vi "AMI_CREA_SECUENCIA_REPITE.vi"(8 "error in (no error)":errorcluster) -> (0 "error out":errorcluster, 1 "Total":string[](array[string]), 2 "Pasos":i32, 3 "Secuencia":string[](array[string]), 4 "Secuciclos":string[](array[string]), 6 "Pasos f":i32)   [LabVIEW 2017]
uses:
  <vilib>/Utility/file.llb/Read Delimited Spreadsheet (string).vi
panel:
  out "idxScanXi":i16
  out "idxScanXf":i16
  out "idxScanYi":i16
  out "idxScanYf":i16
  out "Scan X":bool
  out "Scan Y":bool
  out "idxScanVi":i16
  out "idxScanVf":i16
  out "Scan V":bool
  out "subArray2D":string[][](array[string])
  out "Seq scans":string[](array[string])
  out "Seq final":string[](array[string])
  out "Seq inicial":string[](array[string])
  out "idxScanTi":i16
  out "idxScanZi":i16
  out "idxScanZf":i16
  out "idxScanTf":i16
  out "Array2D":string[][](array[string])
  out "Scan T":bool
  out "Scan Z":bool
  in  "Salir":bool
  in  "Borrar línea":bool
  in  "Grabar":bool
  in  "Cargar":bool
  out "SequenceFile":path
  in  "Añadir: (doble click)":i32(listbox) caption="Válvulas"
  in  "Secuencia":i32(listbox)=-1
  # "Nov 2022 V1.6  a-sslcdms"
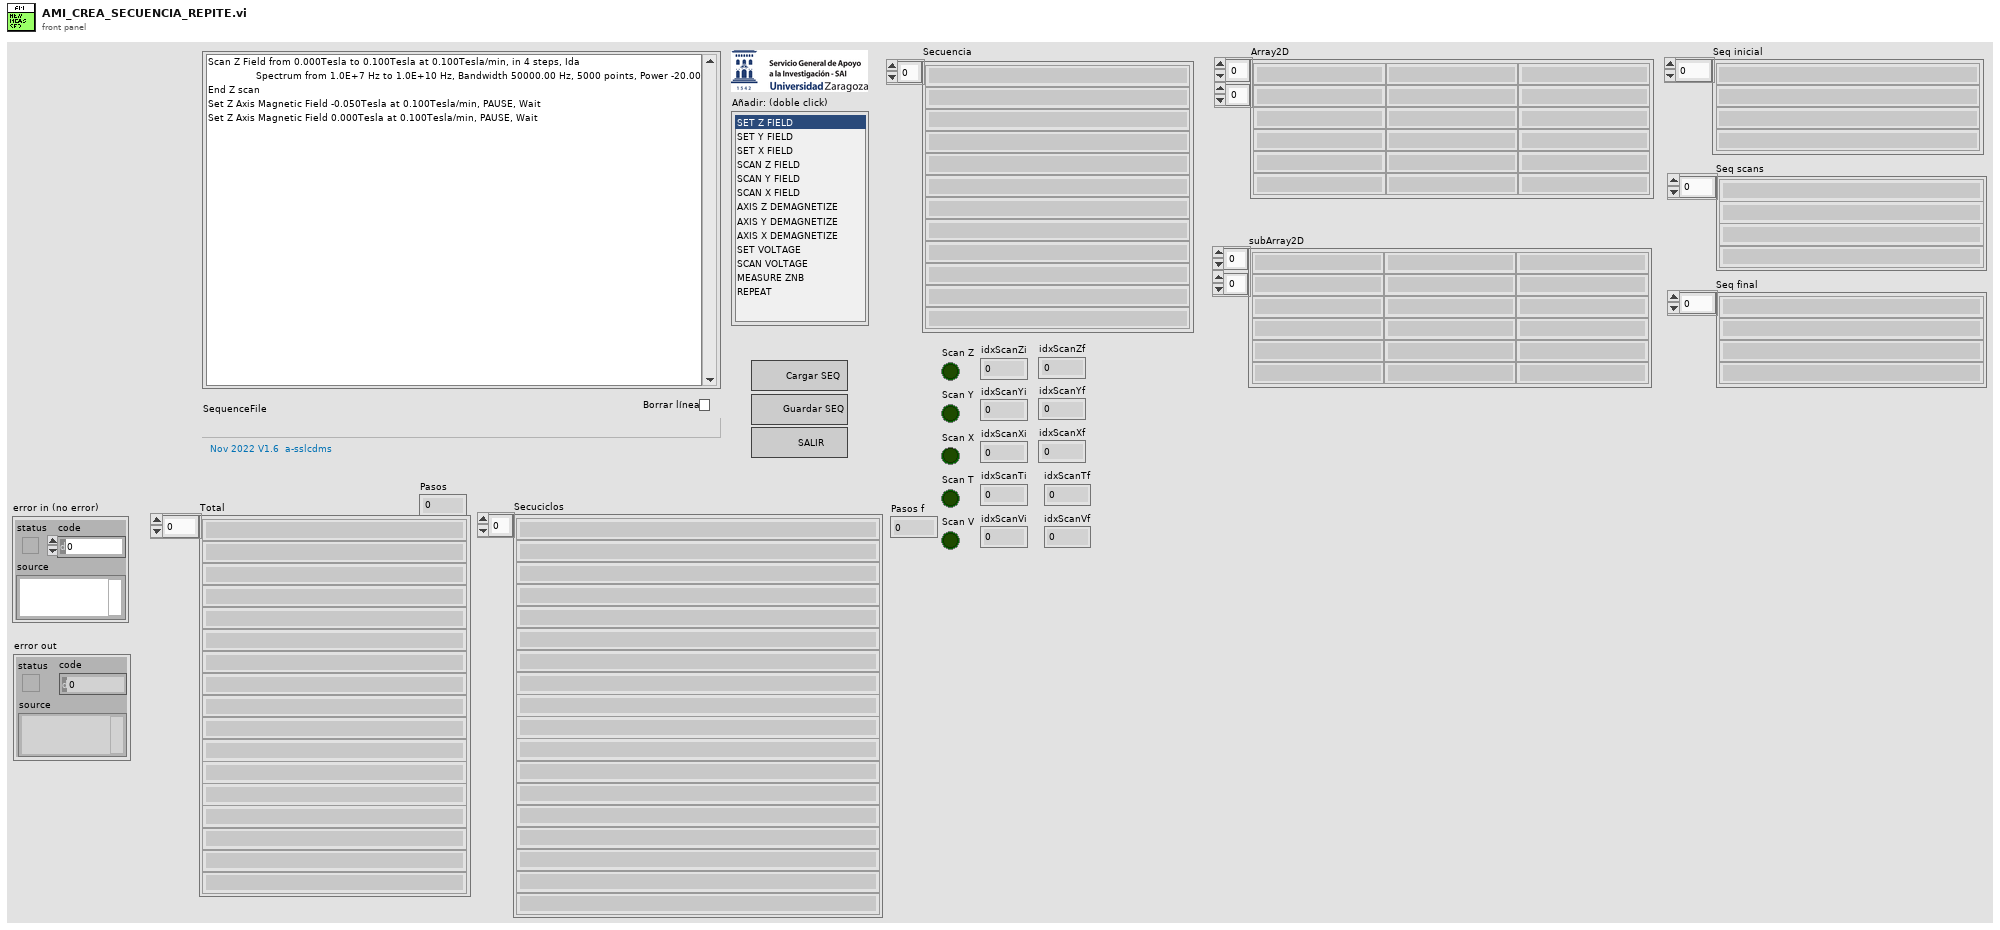
[diagram p1: front panel]
types:
  T1 = enum16{"open", "open or create", "create or replace", "create", "open (read only)"}
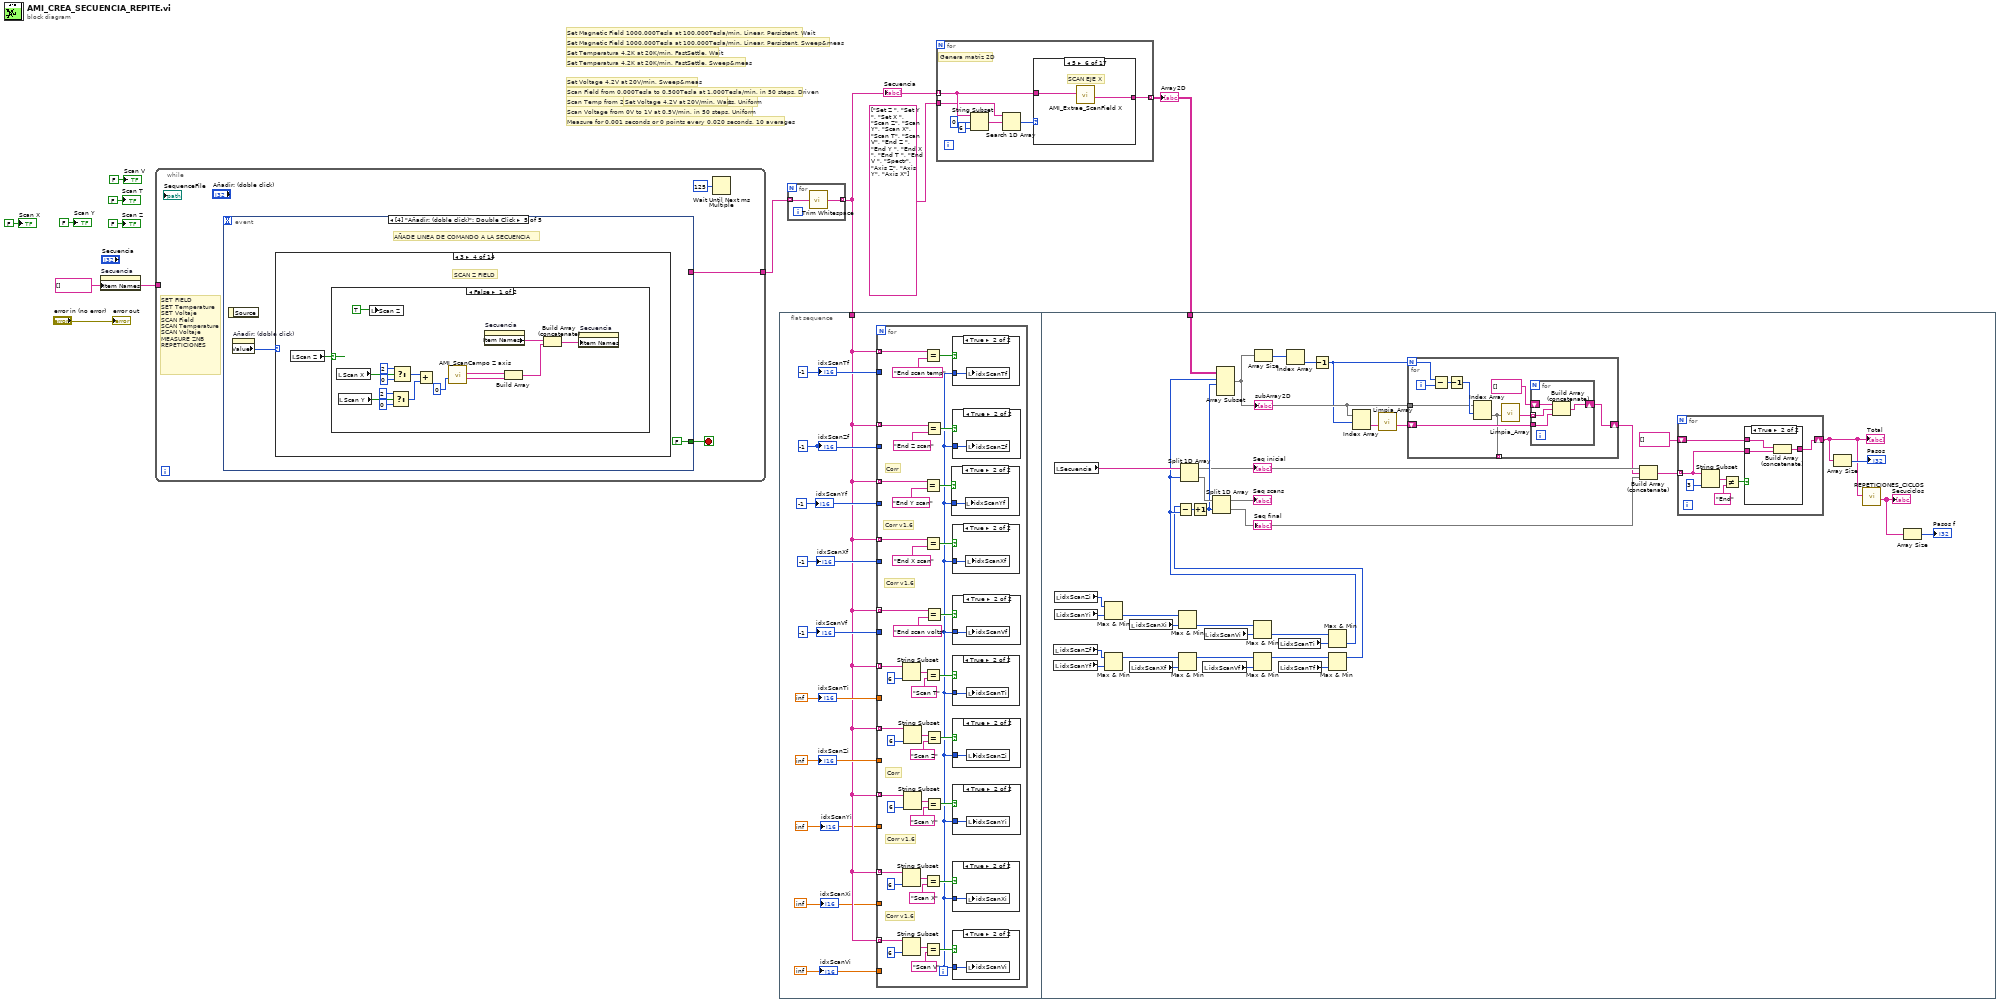
[diagram p0: block diagram]
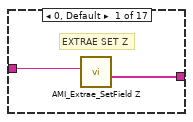
[diagram p13: hidden frame]
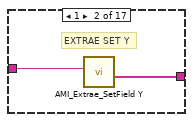
[diagram p14: hidden frame]
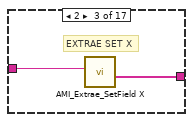
[diagram p15: hidden frame]
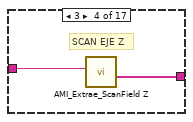
[diagram p16: hidden frame]
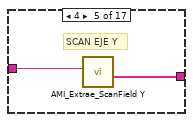
[diagram p17: hidden frame]
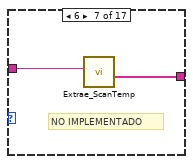
[diagram p18: hidden frame]
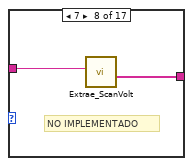
[diagram p19: hidden frame]
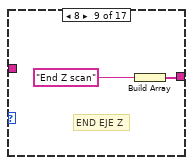
[diagram p20: hidden frame]
diagram:
  w11 = string[] [] ("Item Names")
  # "Measure for 0.001 seconds or 0 points every 0.020 seconds, 10 averages"
  # "Scan Voltage from 0V to 1V at 0.5V/min, in 50 steps, Uniform"
  # "Scan Temp from 20K to 200K at 0.1K/min, in 50 steps, Uniform"
  # "Scan Field from 0.000Tesla to 0.500Tesla at 1.000Tesla/min, in 50 steps, Driven"
  # "Set Temperatura 4.2K at 20K/min, FastSettle, Sweep&meas"
  # "Set Temperatura 4.2K at 20K/min, FastSettle, Wait"
  # "Set Magnetic Field 1000.000Tesla at 100.000Tesla/min, Linear, Persistent, Sweep&meas"
  # "Set Magnetic Field 1000.000Tesla at 100.000Tesla/min, Linear, Persistent, Wait"
  # "Set Voltage 4.2V at 20V/min, Sweep&meas"
  # "Set Voltage 4.2V at 20V/min, Wait"
  n1 = property on="Secuencia" class="LstBox (strict)"("Item Names"=w11) -> ()  [unwired: 2 in, 2 out]
  n2 = while {
    tunnel: w11 -> [_]
    tunnel: [w12] -> w6
    stop <- w13 stop-if-true
    # "SET FIELD\nSET Temperature\nSET Voltaje\nSCAN Field\nSCAN Temperature\nSCAN Voltaje\nMEASURE ZNB\nREPETICIONES"
    n3 = event shown="[4] \"Añadir: (doble click)\": Double Click" {
      selector: _ -> [_ _ _ _ _]
      dyn-events: _ -> [_ _ _ _ _]
      timeout: _ -> [_ _ _ _ _]
      tunnel: [FALSE ("Salir") "Salir" FALSE ("Salir") FALSE ("Salir") FALSE ("Salir")] -> w13
      tunnel: [_ w20 _ _ _] -> w12
      event "Borrar línea": Value Change {
        # "BORRA LA LINEA ACTIVA DE LA SECUENCIA"
        n4 = event-data() -> ()  [unwired: 1 in, 1 out]
        n5 = property on="Secuencia" class="LstBox (strict)"() -> ("Item Names"=w19:string[], "Value"=w18:i32)  [unwired: 2 in, 2 out]
        n6 = Delete From Array(array=w19, length=1, index=w18) -> (array with subset deleted=w16:string[])  [unwired: 1 out]
        n7 = property on="Secuencia" class="LstBox (strict)"("Item Names"=w16) -> ()  [unwired: 2 in, 2 out]
      }
      event "Salir": Value Change {
        # "SALIMOS DEL VI"
        n8 = event-data() -> ()  [unwired: 1 in, 1 out]
        n9 = property on="Secuencia" class="LstBox (strict)"() -> ("Item Names"=w20:string[])  [unwired: 2 in, 2 out]
      }
      event "Cargar": Value Change {
        # "CARGA UNA SECUENCIA ALMACENADA PREVIAMENTE"
        n10 = event-data() -> ()  [unwired: 1 in, 1 out]
        n11 = call-poly <vilib>:"Read Delimited Spreadsheet.vi"() -> ("new file path (Not A Path if cancelled)"=w23:path, "all rows"=w22:string[][])  [unwired: 10 in, 4 out]
        n12 = local write "SequenceFile"(w23) -> ()
        n13 = Index Array(array=w22, index (col)=0 ("disabled index (col)")) -> (element=w24:string[])  [unwired: 1 in]
        n14 = property on="Secuencia" class="LstBox (strict)"("Item Names"=w24) -> ()  [unwired: 2 in, 2 out]
      }
      event "Grabar": Value Change {
        # "GRABA UNA SECUENCIA PARA USAR MAS ADELANTE"
        n15 = event-data() -> ()  [unwired: 1 in, 1 out]
        n16 = property on="Secuencia" class="LstBox (strict)"() -> ("Item Names"=w30:string[])  [unwired: 2 in, 2 out]
        n17 = call <vilib>:"Open_Create_Replace File.vi"("function (open:0)"=T1."create or replace") -> ("new file path"=w27:path)  [unwired: 7 in, 3 out]
        n18 = local write "SequenceFile"(w27) -> ()
        n19 = for {
          tunnel: w30 -> [w33] mode=indexing
          shift-right: [w35] -> _
          shift-left: w27 -> [w36]
          n20 = Concatenate Strings(w33, "\r\n") -> (w32:string)
          n21 = call <vilib>:"Write Characters To File.vi"("append to file? (new file:F)"=TRUE, "character string"=w32, "file path (dialog if empty)"=w36) -> ("new file path (Not A Path if cancelled)"=w35:path)  [unwired: 2 in]
        }
      }
      event "Añadir: (doble click)": Double Click {
        # "AÑADE LINEA DE COMANDO A LA SECUENCIA"
        n22 = event-data() -> ()  [unwired: 1 in, 1 out]
        n23 = property on="Añadir: (doble click)" class="LstBox (strict)"() -> ("Value"=w37:i32)  [unwired: 2 in, 2 out]
        n24 = case shown="3" w37 {
          frame 0, Default {
            # "SET Z FIELD"
            n25 = property on="Secuencia" class="LstBox (strict)"() -> ("Item Names"=w39:string[])  [unwired: 2 in, 2 out]
            n26 = call "AMI_SetCampo Z axis.vi"("Index"=i8 0) -> ("resulting string Z"=w41:string)  [unwired: 7 in, 1 out]
            n27 = Build Array (concatenate)(w39, w41) -> (w40:string[])
            n28 = property on="Secuencia" class="LstBox (strict)"("Item Names"=w40) -> ()  [unwired: 2 in, 2 out]
          }
          frame 1 {
            # "SET Y FIELD"
            n29 = property on="Secuencia" class="LstBox (strict)"() -> ("Item Names"=w44:string[])  [unwired: 2 in, 2 out]
            n30 = call "AMI_SetCampo Y axis.vi"("Index"=i8 0) -> ("resulting string Y"=w46:string)  [unwired: 7 in, 1 out]
            n31 = Build Array (concatenate)(w44, w46) -> (w45:string[])
            n32 = property on="Secuencia" class="LstBox (strict)"("Item Names"=w45) -> ()  [unwired: 2 in, 2 out]
          }
          frame 2 {
            # "SET X FIELD"
            n33 = property on="Secuencia" class="LstBox (strict)"() -> ("Item Names"=w50:string[])  [unwired: 2 in, 2 out]
            n34 = call "AMI_SetCampo X axis.vi"("Index"=i8 0) -> ("resulting string X"=w48:string)  [unwired: 7 in, 1 out]
            n35 = Build Array (concatenate)(w50, w48) -> (w49:string[])
            n36 = property on="Secuencia" class="LstBox (strict)"("Item Names"=w49) -> ()  [unwired: 2 in, 2 out]
          }
          frame 3 {
            # "SCAN Z FIELD"
            n37 = local read "Scan Z"() -> (w51:bool)
            n38 = case shown="False" w51 {
              frame False {
                n39 = local read "Scan X"() -> (w63:bool)
                n40 = local read "Scan Y"() -> (w62:bool)
                n41 = local write "Scan Z"(TRUE ("Scan T")) -> ()
                n42 = Select(t=i8 2 ("Index"), s=w62, f=i8 0 ("Index")) -> (s? t:f=w58:i8)
                n43 = Select(t=i8 2 ("Index"), s=w63, f=i8 0 ("Index")) -> (s? t:f=w59:i8)
                n44 = Add(x=w59, y=w58) -> ()  [unwired: 1 out]
                n45 = call "AMI_ScanCampo Z axis.vi"("Index"=i8 0) -> ("resulting string 2"=w53:string, "resulting string 1"=w52:string)  [unwired: 6 in, 1 out]
                n46 = property on="Secuencia" class="LstBox (strict)"() -> ("Item Names"=w56:string[])  [unwired: 2 in, 2 out]
                n47 = Build Array(w52, w53) -> (w55:string[])
                n48 = Build Array (concatenate)(w56, w55) -> (w54:string[])
                n49 = property on="Secuencia" class="LstBox (strict)"("Item Names"=w54) -> ()  [unwired: 2 in, 2 out]
              }
              frame True {
                n50 = One Button Dialog(message="Solo esta permitido\nun scan de campo por secuencia") -> ()  [unwired: 1 in, 1 out]
              }
            }
          }
          frame 4 {
            # "SCAN Y FIELD"
            n51 = local read "Scan Y"() -> (w68:bool)
            n52 = case shown="False" w68 {
              frame False {
                n53 = local read "Scan X"() -> (w80:bool)
                n54 = local read "Scan Z"() -> (w79:bool)
                n55 = local write "Scan Y"(TRUE ("Scan T")) -> ()
                n56 = Select(t=i8 2 ("Index"), s=w79, f=i8 0 ("Index")) -> (s? t:f=w75:i8)
                n57 = Select(t=i8 2 ("Index"), s=w80, f=i8 0 ("Index")) -> (s? t:f=w76:i8)
                n58 = Add(x=w76, y=w75) -> ()  [unwired: 1 out]
                n59 = call "AMI_ScanCampo Y axis.vi"("Index"=i8 0) -> ("resulting string 2"=w70:string, "resulting string 1"=w69:string)  [unwired: 6 in, 1 out]
                n60 = property on="Secuencia" class="LstBox (strict)"() -> ("Item Names"=w73:string[])  [unwired: 2 in, 2 out]
                n61 = Build Array(w69, w70) -> (w72:string[])
                n62 = Build Array (concatenate)(w73, w72) -> (w71:string[])
                n63 = property on="Secuencia" class="LstBox (strict)"("Item Names"=w71) -> ()  [unwired: 2 in, 2 out]
              }
              frame True {
                n64 = One Button Dialog(message="Solo esta permitido\nun scan de campo por secuencia") -> ()  [unwired: 1 in, 1 out]
              }
            }
          }
          frame 5 {
            # "SCAN X FIELD"
            n65 = local read "Scan X"() -> (w85:bool)
            n66 = case shown="False" w85 {
              frame False {
                n67 = local read "Scan Y"() -> (w97:bool)
                n68 = local read "Scan Z"() -> (w96:bool)
                n69 = local write "Scan X"(TRUE ("Scan T")) -> ()
                n70 = Select(t=i8 2 ("Index"), s=w96, f=i8 0 ("Index")) -> (s? t:f=w92:i8)
                n71 = Select(t=i8 2 ("Index"), s=w97, f=i8 0 ("Index")) -> (s? t:f=w93:i8)
                n72 = Add(x=w93, y=w92) -> ()  [unwired: 1 out]
                n73 = call "AMI_ScanCampo X axis.vi"("Index"=i8 0) -> ("resulting string 2"=w87:string, "resulting string 1"=w86:string)  [unwired: 6 in, 1 out]
                n74 = property on="Secuencia" class="LstBox (strict)"() -> ("Item Names"=w90:string[])  [unwired: 2 in, 2 out]
                n75 = Build Array(w86, w87) -> (w89:string[])
                n76 = Build Array (concatenate)(w90, w89) -> (w88:string[])
                n77 = property on="Secuencia" class="LstBox (strict)"("Item Names"=w88) -> ()  [unwired: 2 in, 2 out]
              }
              frame True {
                n78 = One Button Dialog(message="Solo esta permitido\nun scan de campo por secuencia") -> ()  [unwired: 1 in, 1 out]
              }
            }
          }
          frame 6 {
            # "DESIMANAR Z FIELD"
            n79 = property on="Secuencia" class="LstBox (strict)"() -> ("Item Names"=w102:string[])  [unwired: 2 in, 2 out]
            n80 = call "AMI_Desimana Z axis.vi"("Index"=i8 0) -> ("resulting string Z"=w104:string)  [unwired: 7 in, 1 out]
            n81 = Build Array (concatenate)(w102, w104) -> (w103:string[])
            n82 = property on="Secuencia" class="LstBox (strict)"("Item Names"=w103) -> ()  [unwired: 2 in, 2 out]
          }
          frame 7 {
            # "DESIMANAR Y FIELD"
            n83 = property on="Secuencia" class="LstBox (strict)"() -> ("Item Names"=w107:string[])  [unwired: 2 in, 2 out]
            n84 = call "AMI_Desimana Y axis.vi"("Index"=i8 0) -> ("resulting string Y"=w109:string)  [unwired: 7 in, 1 out]
            n85 = Build Array (concatenate)(w107, w109) -> (w108:string[])
            n86 = property on="Secuencia" class="LstBox (strict)"("Item Names"=w108) -> ()  [unwired: 2 in, 2 out]
          }
          frame 8 {
            # "DESIMANAR X FIELD"
            n87 = property on="Secuencia" class="LstBox (strict)"() -> ("Item Names"=w113:string[])  [unwired: 2 in, 2 out]
            n88 = call "AMI_Desimana X axis.vi"("Index"=i8 0) -> ("resulting string X"=w111:string)  [unwired: 7 in, 1 out]
            n89 = Build Array (concatenate)(w113, w111) -> (w112:string[])
            n90 = property on="Secuencia" class="LstBox (strict)"("Item Names"=w112) -> ()  [unwired: 2 in, 2 out]
          }
          frame 9 {
            # "SET VOLTAGE"
            n91 = case shown="False" FALSE {
              frame False {
                n92 = One Button Dialog(message="Comando desactivado") -> ()  [unwired: 1 in, 1 out]
              }
              frame True {
                n93 = call "PPMS_SetVoltage.vi"("Index"=i8 0) -> ("resulting string 1"=w117:string, "Cancelled?"=w118:bool)  [unwired: 6 in, 1 out]
                n94 = case shown="False" w118 {
                  tunnel: w117 -> [w121 _]
                  frame False {
                    n95 = property on="Secuencia" class="LstBox (strict)"() -> ("Item Names"=w120:string[])  [unwired: 2 in, 2 out]
                    n96 = Build Array (concatenate)(w120, w121) -> (w119:string[])
                    n97 = property on="Secuencia" class="LstBox (strict)"("Item Names"=w119) -> ()  [unwired: 2 in, 2 out]
                  }
                  frame True {
                  }
                }
              }
            }
          }
          frame 10 {
            # "SCAN VOLTAGE"
            n98 = case shown="False" FALSE {
              frame False {
                n99 = One Button Dialog(message="Comando desactivado") -> ()  [unwired: 1 in, 1 out]
              }
              frame True {
                n100 = local read "Scan V"() -> (w124:bool)
                n101 = case shown="False" w124 {
                  frame False {
                    n102 = local read "Scan T"() -> (w132:bool)
                    n103 = local read "Scan Z"() -> (w133:bool)
                    n104 = local write "Scan V"(TRUE ("Scan T")) -> ()
                    n105 = Select(t=i8 2 ("Index"), s=w132, f=i8 0 ("Index")) -> (s? t:f=w130:i8)
                    n106 = Select(t=i8 2 ("Index"), s=w133, f=i8 0 ("Index")) -> (s? t:f=w131:i8)
                    n107 = Add(x=w131, y=w130) -> ()  [unwired: 1 out]
                    n108 = call "PPMS_ScanVoltage.vi"("Index"=i8 0) -> ("resulting string 2"=w135:string, "resulting string 1"=w136:string, "Cancelled?"=w137:bool)  [unwired: 5 in, 1 out]
                    n109 = case shown="False" w137 {
                      tunnel: w136 -> [w142 _]
                      tunnel: w135 -> [w141 _]
                      frame False {
                        n110 = property on="Secuencia" class="LstBox (strict)"() -> ("Item Names"=w140:string[])  [unwired: 2 in, 2 out]
                        n111 = Build Array(w142, w141) -> (w139:string[])
                        n112 = Build Array (concatenate)(w140, w139) -> (w138:string[])
                        n113 = property on="Secuencia" class="LstBox (strict)"("Item Names"=w138) -> ()  [unwired: 2 in, 2 out]
                      }
                      frame True {
                      }
                    }
                  }
                  frame True {
                    n114 = One Button Dialog(message="Solo esta permitido\nun scan de temperatura por secuencia") -> ()  [unwired: 1 in, 1 out]
                  }
                }
              }
            }
          }
          frame 11 {
            # "MEASURE CASE  Analizador de frecuencias"
            n115 = local read "Scan Z"() -> (w148:bool)
            n116 = local read "Scan Y"() -> (w155:bool)
            n117 = local read "Scan Z"() -> (w156:bool)
            n118 = Select(t=i8 2 ("Index"), s=w148, f=i8 0 ("Index")) -> (s? t:f=w147:i8)
            n119 = Select(t=i8 2 ("Index"), s=w155, f=i8 0 ("Index")) -> (s? t:f=w151:i8)
            n120 = Select(t=i8 2 ("Index"), s=w156, f=i8 0 ("Index")) -> (s? t:f=w152:i8)
            n121 = Compound Arithmetic op=ADD(w152, w151, w147) -> (w146:i8)
            n122 = call "PPMS_FreqMeas.vi"("Index"=w146) -> ("resulting string 1"=w144:string, "Cancelled?"=w145:bool)  [unwired: 5 in, 2 out]
            n123 = case shown="False" w145 {
              tunnel: w144 -> [w162 _]
              frame False {
                n124 = property on="Secuencia" class="LstBox (strict)"() -> ("Item Names"=w160:string[])  [unwired: 2 in, 2 out]
                n125 = Build Array(w162) -> (w159:string[])
                n126 = Build Array (concatenate)(w160, w159) -> (w161:string[])
                n127 = property on="Secuencia" class="LstBox (strict)"("Item Names"=w161) -> ()  [unwired: 2 in, 2 out]
              }
              frame True {
              }
            }
          }
          frame 12 {
            n128 = call "PPMS_Repeticiones.vi"() -> ("Ciclos"=w164:i32, "Cancelled?"=w163:bool)  [unwired: 10 in]
            n129 = Format Into String(format string="%s %d %s", "Repetir: " ("input 1"), w164, " veces" ("input 3")) -> (resulting string=w169:string)  [unwired: 2 in, 1 out]
            n130 = case shown="False" w163 {
              tunnel: w169 -> [w173 _]
              tunnel: "Fin repeticiones" ("input 1") -> [w172 _]
              frame False {
                n131 = property on="Secuencia" class="LstBox (strict)"() -> ("Item Names"=w171:string[])  [unwired: 2 in, 2 out]
                n132 = Build Array (concatenate)(w171, w173, w172) -> (w170:string[])
                n133 = property on="Secuencia" class="LstBox (strict)"("Item Names"=w170) -> ()  [unwired: 2 in, 2 out]
              }
              frame True {
              }
            }
          }
          frame 13 {
            # "End Program"
            n134 = property on="Secuencia" class="LstBox (strict)"() -> ("Item Names"=w174:string[])  [unwired: 2 in, 2 out]
            n135 = Build Array (concatenate)(w174, "End Program" ("message")) -> ()  [unwired: 1 out]
            n136 = property on="Secuencia" class="LstBox (strict)"("Item Names"=w174) -> ()  [unwired: 2 in, 2 out]
          }
        }
      }
    }
    n137 = Wait Until Next ms Multiple(millisecond multiple=u32 125) -> ()  [unwired: 1 out]
  }
  n138 = flat-sequence {
    tunnel: w5 -> [w178]
    tunnel: w4 -> [w268]
    frame #0 {
      w177 = inf
      w176 = inf
      w180 = i16 -1 ("idxScanT")
      w179 = i16 -1 ("idxScanT")
      w182 = i16 -1 ("idxScanT")
      w181 = inf
      w183 = inf
      w184 = inf
      w185 = i16 -1 ("idxScanT")
      w186 = i16 -1 ("idxScanT")
      n139 = for {
        tunnel: w178 -> [w218] mode=indexing
        tunnel: w186 -> [_]
        tunnel: w178 -> [w217] mode=indexing
        tunnel: w185 -> [_]
        tunnel: w178 -> [w215] mode=indexing
        tunnel: w178 -> [w214] mode=indexing
        tunnel: w183 -> [_]
        tunnel: w184 -> [_]
        tunnel: w178 -> [w210] mode=indexing
        tunnel: w181 -> [_]
        tunnel: w178 -> [w206] mode=indexing
        tunnel: w182 -> [_]
        tunnel: w178 -> [w203] mode=indexing
        tunnel: w179 -> [_]
        tunnel: w178 -> [w198] mode=indexing
        tunnel: w180 -> [_]
        tunnel: w178 -> [w196] mode=indexing
        tunnel: w176 -> [_]
        tunnel: w178 -> [w189] mode=indexing
        tunnel: w177 -> [_]
        i -> [w187]
        # "Corr v1.6"
        # "Corr v1.6"
        # "Corr v1.6"
        # "Corr v1.6"
        # "Corr"
        # "Corr"
        n140 = String Subset(string=w215, length (rest)=6 ("length (rest)")) -> (substring=w212:string)  [unwired: 1 in]
        n141 = String Subset(string=w189, length (rest)=6 ("length (rest)")) -> (substring=w188:string)  [unwired: 1 in]
        n142 = String Subset(string=w210, length (rest)=6 ("length (rest)")) -> (substring=w211:string)  [unwired: 1 in]
        n143 = String Subset(string=w214, length (rest)=6 ("length (rest)")) -> (substring=w213:string)  [unwired: 1 in]
        n144 = String Subset(string=w196, length (rest)=6 ("length (rest)")) -> (substring=w197:string)  [unwired: 1 in]
        n145 = Equal?(x=w203, y="End Y scan" ("trimmed string")) -> (x = y?=w201:bool)
        n146 = Equal?(x=w218, y="End scan temp" ("trimmed string")) -> (x = y?=w226:bool)
        n147 = Equal?(x=w198, y="End X scan" ("trimmed string")) -> (x = y?=w200:bool)
        n148 = Equal?(x=w212, y="Scan T" ("trimmed string")) -> (x = y?=w221:bool)
        n149 = Equal?(x=w188, y="Scan X" ("trimmed string")) -> (x = y?=w191:bool)
        n150 = Equal?(x=w211, y="Scan V" ("trimmed string")) -> (x = y?=w208:bool)
        n151 = Equal?(x=w217, y="End Z scan" ("trimmed string")) -> (x = y?=w225:bool)
        n152 = Equal?(x=w206, y="End scan volts" ("trimmed string")) -> (x = y?=w204:bool)
        n153 = Equal?(x=w213, y="Scan Z" ("trimmed string")) -> (x = y?=w222:bool)
        n154 = Equal?(x=w197, y="Scan Y" ("trimmed string")) -> (x = y?=w194:bool)
        n155 = case shown="True" w201 {
          tunnel: w187 -> [_ w231]
          frame False {
          }
          frame True {
            n156 = local write "idxScanYf"(w231) -> ()
          }
        }
        n157 = case shown="True" w226 {
          tunnel: w187 -> [_ w237]
          frame False {
          }
          frame True {
            n158 = local write "idxScanTf"(w237) -> ()
          }
        }
        n159 = case shown="True" w200 {
          tunnel: w187 -> [_ w230]
          frame False {
          }
          frame True {
            n160 = local write "idxScanXf"(w230) -> ()
          }
        }
        n161 = case shown="True" w221 {
          tunnel: w187 -> [_ w235]
          frame False {
          }
          frame True {
            n162 = local write "idxScanTi"(w235) -> ()
          }
        }
        n163 = case shown="True" w191 {
          tunnel: w187 -> [_ w228]
          frame False {
          }
          frame True {
            n164 = local write "idxScanXi"(w228) -> ()
          }
        }
        n165 = case shown="True" w208 {
          tunnel: w187 -> [_ w233]
          frame False {
          }
          frame True {
            n166 = local write "idxScanVi"(w233) -> ()
          }
        }
        n167 = case shown="True" w225 {
          tunnel: w187 -> [_ w236]
          frame False {
          }
          frame True {
            n168 = local write "idxScanZf"(w236) -> ()
          }
        }
        n169 = case shown="True" w204 {
          tunnel: w187 -> [_ w232]
          frame False {
          }
          frame True {
            n170 = local write "idxScanVf"(w232) -> ()
          }
        }
        n171 = case shown="True" w222 {
          tunnel: w187 -> [_ w234]
          frame False {
          }
          frame True {
            n172 = local write "idxScanZi"(w234) -> ()
          }
        }
        n173 = case shown="True" w194 {
          tunnel: w187 -> [_ w229]
          frame False {
          }
          frame True {
            n174 = local write "idxScanYi"(w229) -> ()
          }
        }
      }
      "idxScanTf" <- w186
      "idxScanZf" <- w185
      "idxScanTi" <- w184
      "idxScanZi" <- w183
      "idxScanVf" <- w182
      "idxScanVi" <- w181
      "idxScanYf" <- w179
      "idxScanXf" <- w180
      "idxScanYi" <- w176
      "idxScanXi" <- w177
    }
    frame #1 {
      n175 = local read "idxScanZf"() -> (w272:i16)
      n176 = local read "idxScanYf"() -> (w273:i16)
      n177 = local read "Secuencia"() -> (w276:string[])
      n178 = local read "idxScanZi"() -> (w275:i16)
      n179 = local read "idxScanYi"() -> (w274:i16)
      n180 = Max & Min(x=w275, y=w274) -> (min(x,y)=w252:i16)  [unwired: 1 out]
      n181 = Max & Min(x=w272, y=w273) -> (max(x,y)=w251:i16)  [unwired: 1 out]
      n182 = local read "idxScanXf"() -> (w254:i16)
      n183 = local read "idxScanXi"() -> (w253:i16)
      n184 = Max & Min(x=w252, y=w253) -> (min(x,y)=w242:i16)  [unwired: 1 out]
      n185 = Max & Min(x=w251, y=w254) -> (max(x,y)=w240:i16)  [unwired: 1 out]
      n186 = local read "idxScanVf"() -> (w246:i16)
      n187 = local read "idxScanVi"() -> (w247:i16)
      n188 = Max & Min(x=w242, y=w247) -> (min(x,y)=w243:i16)  [unwired: 1 out]
      n189 = Max & Min(x=w240, y=w246) -> (max(x,y)=w238:i16)  [unwired: 1 out]
      n190 = local read "idxScanTi"() -> (w244:i16)
      n191 = local read "idxScanTf"() -> (w245:i16)
      n192 = Max & Min(x=w243, y=w244) -> (min(x,y)=w241:i16)  [unwired: 1 out]
      n193 = Split 1D Array(array=w276, index=w241) -> (first subarray=w259:string[], second subarray=w270:string[])
      "Seq inicial" <- w259
      n194 = Max & Min(x=w238, y=w245) -> (max(x,y)=w239:i16)  [unwired: 1 out]
      n195 = Subtract(x=w239, y=w241) -> (x-y=w269:i16)
      n196 = Increment(x=w269) -> (x+1=w267:i16)
      n197 = Split 1D Array(array=w270, index=w267) -> (first subarray=→"Seq scans":string[], second subarray=w260:string[])
      "Seq final" <- w260
      n198 = Array Subset(array=w268, index (row)=w241, length (row)=w267) -> (w264:string[][])  [unwired: 2 in]
      "subArray2D" <- w264
      n199 = Array Size(array=w264) -> (size(s)=w263:i32[])
      n200 = Index Array(array=w263) -> (element=w262:i32)  [unwired: 1 in]
      n201 = Decrement(x=w262) -> (x-1=w261:i32)
      n202 = Index Array(array=w264, index (row)=w261) -> (element=w265:string[])  [unwired: 1 in]
      n203 = call "Limpia_Array.vi"("Array in"=w265) -> ("Array out"=w266:string[])  [unwired: 10 in]
      n204 = for {
        N: w261 -> [w297]
        tunnel: w264 -> [w294]
        shift-right: [w290] -> w258
        shift-left: w266 -> [w291]
        tunnel: [w288] -> _ mode=indexing
        i -> [w296]
        n205 = Subtract(x=w297, y=w296) -> (x-y=w293:i32)
        n206 = Decrement(x=w293) -> (x-1=w295:i32)
        n207 = Index Array(array=w294, index (row)=w295) -> (element=w288:string[])  [unwired: 1 in]
        n208 = call "Limpia_Array.vi"("Array in"=w288) -> ("Array out"=w289:string[])  [unwired: 10 in]
        n209 = for {
          tunnel: w289 -> [w300] mode=indexing
          shift-right: [w298] -> w290
          shift-left: string[] [] -> [w301]
          tunnel: w291 -> [w299]
          n210 = Build Array (concatenate)(w301, w300, w299) -> (w298:string[])
        }
      }
      n211 = Build Array (concatenate)(w259, w258, w260) -> (w257:string[])
      n212 = for {
        tunnel: w257 -> [w277] mode=indexing
        shift-right: [w279] -> w250
        shift-left: string[] [] -> [w280]
        n213 = String Subset(string=w277, length (rest)=3 ("length (rest)")) -> (substring=w283:string)  [unwired: 1 in]
        n214 = Not Equal?(x=w283, y="End" ("trimmed string")) -> (x != y?=w278:bool)
        n215 = case shown="True" w278 {
          tunnel: w280 -> [w284 w287]
          tunnel: [w284 w286] -> w279
          tunnel: w277 -> [_ w285]
          frame False {
          }
          frame True {
            n216 = Build Array (concatenate)(w287, w285) -> (w286:string[])
          }
        }
      }
      "Total" <- w250
      n217 = Array Size(array=w250) -> (size(s)=→"Pasos":i32)
      n218 = call "REPETICIONES_CICLOS.vi"("Secuencia"=w250) -> ("Secuciclos"=w249:string[])  [unwired: 9 in, 1 out]
      "Secuciclos" <- w249
      n219 = Array Size(array=w249) -> (size(s)=→"Pasos f":i32)
    }
  }
  n220 = for {
    tunnel: w6 -> [w303] mode=indexing
    tunnel: [w302] -> w5 mode=indexing
    n221 = call <vilib>:"Trim Whitespace.vi"("string"=w303) -> ("trimmed string"=w302:string)  [unwired: 1 in]
  }
  "Secuencia" <- w5
  n222 = for {
    tunnel: w5 -> [w306] mode=indexing
    tunnel: [w304] -> w4 mode=indexing
    tunnel: string[] ["Set Z ", "Set Y ", "Set X ", "Scan Z", "Scan Y", "Scan X", "Scan T", "Scan V", "End Z ", "End Y ", "End X ", "End T ", "End V ", "Spectr", "Axis Z", "Axis Y", "Axis X"] ("Array") -> [w305]
    # "Genera matriz 2D"
    n223 = String Subset(string=w306, offset (0)=0, length (rest)=6 ("length (rest)")) -> (substring=w308:string)
    n224 = Search 1D Array(1D array=w305, element=w308) -> (index of element=w307:i32)  [unwired: 1 in]
    n225 = case shown="5" w307 {
      tunnel: w306 -> [w312 w314 w316 w318 w320 w322 w324 w326 _ _ _ _ _ w338 w340 w342 w344]
      tunnel: [w311 w313 w315 w317 w319 w321 w323 w325 w327 w329 w331 w333 w335 w337 w339 w341 w343] -> w304
      frame 0, Default {
        # "EXTRAE SET Z"
        n226 = call "AMI_Extrae_SetField Z.vi"("String"=w312) -> ("Array"=w311:string[])  [unwired: 10 in]
      }
      frame 1 {
        # "EXTRAE SET Y"
        n227 = call "AMI_Extrae_SetField Y.vi"("String"=w314) -> ("Array"=w313:string[])  [unwired: 10 in]
      }
      frame 2 {
        # "EXTRAE SET X"
        n228 = call "AMI_Extrae_SetField X.vi"("String"=w316) -> ("Array"=w315:string[])  [unwired: 10 in]
      }
      frame 3 {
        # "SCAN EJE Z"
        n229 = call "AMI_Extrae_ScanField Z.vi"("F string"=w318) -> ("Array F"=w317:string[])  [unwired: 10 in]
      }
      frame 4 {
        # "SCAN EJE Y"
        n230 = call "AMI_Extrae_ScanField Y.vi"("F string"=w320) -> ("Array F"=w319:string[])  [unwired: 10 in]
      }
      frame 5 {
        # "SCAN EJE X"
        n231 = call "AMI_Extrae_ScanField X.vi"("F string"=w322) -> ("Array F"=w321:string[])  [unwired: 10 in]
      }
      frame 6 {
        # "NO IMPLEMENTADO"
        n232 = call "Extrae_ScanTemp.vi"("T string"=w324) -> ("Array T"=w323:string[])  [unwired: 10 in]
      }
      frame 7 {
        # "NO IMPLEMENTADO"
        n233 = call "Extrae_ScanVolt.vi"("V string"=w326) -> ("Array V"=w325:string[])  [unwired: 10 in]
      }
      frame 8 {
        # "END EJE Z"
        n234 = Build Array("End Z scan" ("trimmed string")) -> (w327:string[])
      }
      frame 9 {
        # "END EJE Y"
        # "End scan temp"
        n235 = Build Array("End Y scan" ("trimmed string")) -> (w329:string[])
      }
      frame 10 {
        # "END EJE X"
        # "End scan temp"
        n236 = Build Array("End X scan" ("trimmed string")) -> (w331:string[])
      }
      frame 11 {
        # "NO IMPLEMENTADO"
        # "End scan temp"
        n237 = Build Array("End T scan" ("trimmed string")) -> (w333:string[])
      }
      frame 12 {
        # "NO IMPLEMENTADO"
        # "End scan temp"
        n238 = Build Array("End V scan" ("trimmed string")) -> (w335:string[])
      }
      frame 13 {
        # "EXTRAE MEDIDA ZNB"
        n239 = call "AMI_Extrae_ZNB_Measure.vi"("String"=w338) -> ("Array"=w337:string[])  [unwired: 10 in]
      }
      frame 14 {
        # "DESIMANAR EJE Z"
        n240 = call "AMI_Extrae_ZNB_Measure.vi"("String"=w340) -> ("Array"=w339:string[])  [unwired: 10 in]
      }
      frame 15 {
        # "DESIMANAR EJE Y"
        n241 = call "AMI_Extrae_ZNB_Measure.vi"("String"=w342) -> ("Array"=w341:string[])  [unwired: 10 in]
      }
      frame 16 {
        # "DESIMANAR EJE X"
        n242 = call "AMI_Extrae_ZNB_Measure.vi"("String"=w344) -> ("Array"=w343:string[])  [unwired: 10 in]
      }
    }
  }
  "Array2D" <- w4
  "error out" <- "error in (no error)"
  "Scan Z" <- FALSE ("Loop H")
  "Scan T" <- FALSE ("Loop T")
  "Scan V" <- FALSE ("Loop T")
  "Scan Y" <- FALSE ("Loop H")
  "Scan X" <- FALSE ("Loop H")
